vi "unpack_rm_depth_ahat.vi"(11 "payload":u64) -> (0 "error":bool, 1 "metadata":cluster{"sensor_ticks":u64}, 2 "ab":u16[][](array[numeric]), 3 "depth":u16[][](array[numeric]))   [LabVIEW 2023]
panel:
  in  "rm_depth_ahat_metadata":cluster{"sensor_ticks":u64}
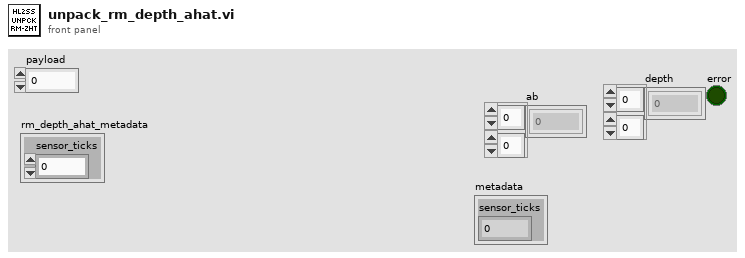
[diagram p1: front panel]
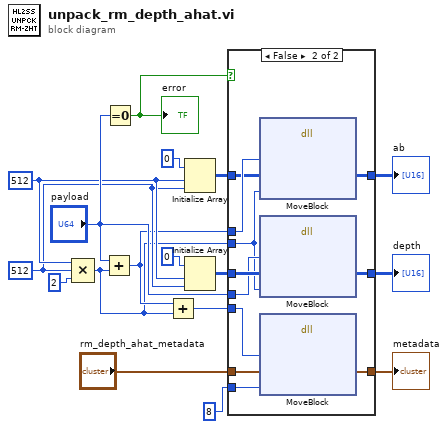
[diagram p0: block diagram]
diagram:
  w4 = u16 512 ("value")
  w5 = u16 512 ("value")
  n1 = Compound Arithmetic op=MULTIPLY(w5, w4, u64 2 ("value")) -> (w2:u64)
  n2 = Add(x="payload", y=w2) -> (x+y=w3:u64)
  n3 = Equal To 0?(x="payload") -> (x = 0?=w10:bool)
  "error" <- w10
  n4 = Add(x=w3, y=w2) -> (x+y=w1:u64)
  n5 = Initialize Array(u16 0, w5, w4) -> (w6:u16[][])
  n6 = Initialize Array(u16 0, w5, w4) -> (w15:u16[][])
  n7 = case shown="False" w10 {
    tunnel: w15 -> [w20 w31]
    tunnel: "payload" -> [_ w30]
    tunnel: w2 -> [_ w21]
    tunnel: w3 -> [_ w24]
    tunnel: u64 8 ("size") -> [_ w29]
    tunnel: "rm_depth_ahat_metadata" -> [w19 w28]
    tunnel: [w20 w27] -> w12
    tunnel: [w19 w26] -> w9
    tunnel: [w18 w25] -> w8
    tunnel: w6 -> [w18 w23]
    tunnel: w1 -> [_ w22]
    frame True {
    }
    frame False {
      n8 = dll-call lib="LabVIEW" fn="MoveBlock"("ps"=w24, "pd"=w23, "size"=w21) -> ("pd"=w25:u16[][])  [unwired: 6 in, 2 out]
      n9 = dll-call lib="LabVIEW" fn="MoveBlock"("ps"=w30, "pd"=w31, "size"=w21) -> ("pd"=w27:u16[][])  [unwired: 6 in, 2 out]
      n10 = dll-call lib="LabVIEW" fn="MoveBlock"("ps"=w22, "pd"=w28, "size"=w29) -> ("pd"=w26:cluster{"sensor_ticks":u64})  [unwired: 6 in, 2 out]
    }
  }
  "depth" <- w12
  "metadata" <- w9
  "ab" <- w8
